vi "test filter 1d array.vi"() -> ()   [LabVIEW 2017]
uses:
  37b0788e-76bc-4745-a657-81b310b30fe1.vi
  3e4efcde-7aa0-4698-9165-9e23cdf67ab6.vi
  37b0788e-76bc-4745-a657-81b310b30fe1.vi/eb2405bd-5b2e-436b-9bb3-692ecf4a9268.vi
  37b0788e-76bc-4745-a657-81b310b30fe1.vi/c8ad12e3-5e6d-40e1-92e0-1426ef45ec41.vi
  37b0788e-76bc-4745-a657-81b310b30fe1.vi/effcbc1a-e97c-42d4-b61f-d821de102707.vi
  3e4efcde-7aa0-4698-9165-9e23cdf67ab6.vi/eb2405bd-5b2e-436b-9bb3-692ecf4a9268.vi
  3e4efcde-7aa0-4698-9165-9e23cdf67ab6.vi/c8ad12e3-5e6d-40e1-92e0-1426ef45ec41.vi
  3e4efcde-7aa0-4698-9165-9e23cdf67ab6.vi/effcbc1a-e97c-42d4-b61f-d821de102707.vi
panel:
  out "filtered array":string[](array[string])
  out "filtered array":string[](array[string])
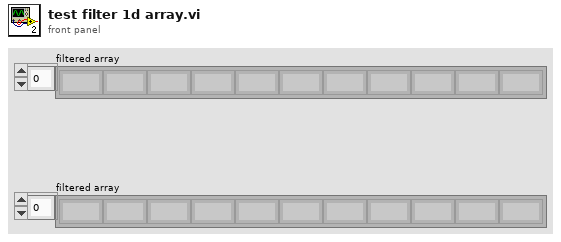
[diagram p1: front panel]
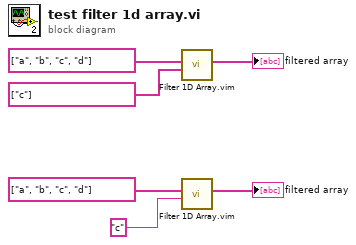
[diagram p0: block diagram]
diagram:
  n1 = call "Filter 1D Array.vim"("items to filter"=string[] ["c"], "array"=string[] ["a", "b", "c", "d"]) -> ("filtered array"=→"filtered array":string[])  [unwired: 4 in, 1 out]
  n2 = call "Filter 1D Array.vim"("items to filter"="c" ("String"), "array"=string[] ["a", "b", "c", "d"]) -> ("filtered array"=→"filtered array":string[])  [unwired: 4 in, 1 out]
